vi "Read Continuous Data and Write to Shared Variable.vi"(8 "error in":errorcluster) -> (0 "error out":errorcluster)   [LabVIEW 2017, in "DTACQ - Network Enabled Device Driver.lvlib"]
doc: "Captures a single buffer length of data and publishes that data through shared variables."
uses:
  DTACQ - Network Enabled Device Driver.lvlib
  FGV Operaions--Enum.ctl
  Network Shared Variables/Typedefs/X and Y Variant Arrays--Cluster.ctl
  Communications/Communications Library.lvlib
  Network Shared Variables/Shared Variables Library.lvlib
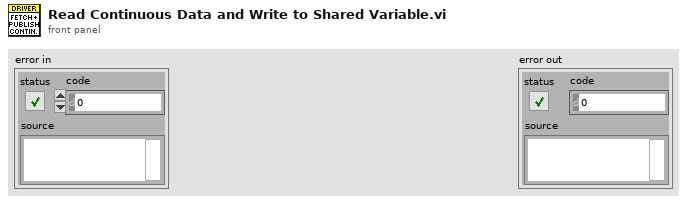
[diagram p1: front panel]
types:
  T1 = typedef "DTACQ - Network Enabled Device Driver.lvlib/FGV Operaions--Enum.ctl" = enum16{"Get Driver Settings", "Set Driver Settings", "Search Variable Names", "Close Connections", "Open Connections", "Get Variable References", "Set Variable References", "Clear"}
  T2 = typedef "DTACQ - Network Enabled Device Driver.lvlib/Driver Global Settings--Typedef.ctl" = cluster{"Waveform Length":i32, "Data Size":T3, "DTACQ Connection Data":T4}
  T3 = typedef "Communications Library.lvlib/Data Size--Enum.ctl" = enum16{"16 Bit (Signed Short)", "32 Bit (Signed Long)"}
  T4 = typedef "Communications Library.lvlib/DTACQ Connection Data--Cluster.ctl" = cluster{"Description":string, "Address":string, "Port":u16, "timeout (ms)":i32, "Termination Character":string, "TCP Connection Reference":refnum<k5>, "Open Connection":bool}
  T5 = typedef "Communications Library.lvlib/DTACQ Module Configuration--Cluster.ctl" = cluster{"Name":string, "Position":string, "Module Type":T6, "Control Port":i32, "Timeout (ms)":i32, "Channels":i32}
  T6 = typedef "Communications Library.lvlib/DTACQ Device Type--Enum.ctl" = enum16{"Carrier", "Analog In Module", "Analog Out Module", "Generic Module"}
  T7 = typedef "Shared Variables Library.lvlib/X and Y Variant Arrays--Cluster.ctl" = cluster{"X-Data":variant[], "Y-Data":variant[]}
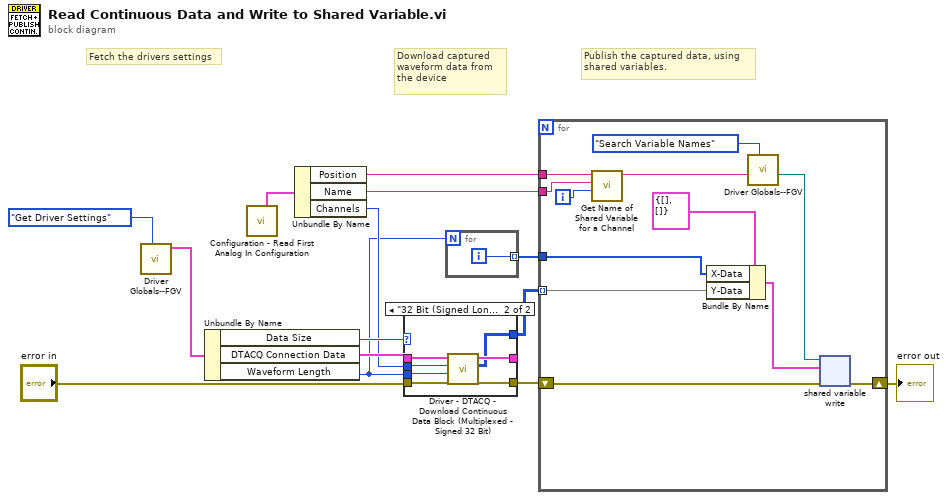
[diagram p0: block diagram]
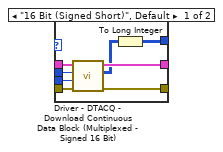
[diagram p2: hidden frame]
diagram:
  # "Publish the captured data, using\nshared variables."
  # "Download captured\nwaveform data from\nthe device"
  # "Fetch the drivers settings"
  n1 = call "Driver Globals--FGV.vi"(7:FGV_Operaions--Enum."Get Driver Settings") -> ("Driver Settings Out"=w13:T2)  [unwired: 7 in, 3 out]
  n2 = Unbundle By Name(w13) -> ("Data Size"=w11:T3, "DTACQ Connection Data"=w10:T4, "Waveform Length"=w7:i32)
  n3 = call "Configuration - Read First Analog In Configuration.vi"() -> ("AI - Module Configuration"=w12:T5)  [unwired: 7 in, 4 out]
  n4 = Unbundle By Name(w12) -> ("Position"=w2:string, "Name"=w1:string, "Channels"=w9:i32)
  n5 = case shown="\"32 Bit (Signed Long)\"" w11 {
    tunnel: "error in" -> [w22 w29]
    tunnel: w10 -> [w21 w28]
    tunnel: [w20 w25] -> _
    tunnel: [w16 w23] -> w5
    tunnel: w7 -> [w19 w26]
    tunnel: w9 -> [w18 w27]
    tunnel: [w17 w24] -> w6
    frame "16 Bit (Signed Short)", Default {
      n6 = call "Driver - DTACQ - Download Continuous Data Block (Multiplexed - Signed 16 Bit).vi"("error in"=w22, "Number of Samples"=w19, "Number of Channels"=w18, "DTACQ Connection Data In"=w21) -> ("error out"=w17:errorcluster, "Data"=w15:i16[][], "DTACQ Connection Data Out"=w20:T4)  [unwired: 4 in, 1 out]
      n7 = To Long Integer(number=w15) -> (32bit integer=w16:i32[][])
    }
    frame "32 Bit (Signed Long)" {
      n8 = call "Driver - DTACQ - Download Continuous Data Block (Multiplexed - Signed 32 Bit).vi"("error in"=w29, "Number of Samples"=w26, "Number of Channels"=w27, "DTACQ Connection Data In"=w28) -> ("error out"=w24:errorcluster, "Data"=w23:i32[][], "DTACQ Connection Data Out"=w25:T4)  [unwired: 4 in, 1 out]
    }
  }
  n9 = for {
    N: w7 -> [_]
    tunnel: [w30] -> w8 mode=indexing
    i -> [w30]
  }
  n10 = for {
    tunnel: w5 -> [w41] mode=indexing
    tunnel: w8 -> [w40]
    tunnel: w2 -> [w39]
    tunnel: w1 -> [w38]
    shift-right: [w31] -> w3
    shift-left: w6 -> [w32]
    i -> [w42]
    n11 = call "Get Name of Shared Variable for a Channel.vi"("Channel Number"=w42, "Module Name"=w38, "Module Position"=w39) -> ("Shared Variable Name"=w35:string)  [unwired: 8 in]
    n12 = Bundle By Name(cluster=T7 {"X-Data"=[], "Y-Data"=[]} ("Data Cluster"), "X-Data"=w40, "Y-Data"=w41) -> (w33:T7)
    n13 = call "Driver Globals--FGV.vi"(7:FGV_Operaions--Enum."Search Variable Names", "Name"=w35) -> ("Searched Reference"=w34:refnum<k21>)  [unwired: 6 in, 3 out]
    n14 = shared-variable-write(w34, w32, w33) -> (w31:errorcluster)  [unwired: 1 out]
  }
  "error out" <- w3
